vi "CalibrateImage.vi"() -> ()   [LabVIEW 2009]
uses:
  <vilib>/vision/NI_Vision_Development_Module.lvlib
panel:
  in  "Interpolation Type":u32(ring) items=["Zero Order", "Bi-Linear", "Quadratic", "Cubic Spline"]
  out "'input Image 2":T1(plugin-control)
  in  "Grid Descriptor":T2={"X Step"=1.0, "Y Step"=1.0, "Unit"=enum."Undefined", "Threshold Range"={"Lower value"=30.0, "Upper value"=96.0}} {"Threshold Range"."Upper value" format="%.2f"; "Threshold Range"."Lower value" format="%.2f"; "Y Step" format="%.2f"; "X Step" format="%.2f"}
  in  "Calibration Learn Setup":T4={"Distortion"=0, "Corrected Image Scaling"=0, "Corrected Image Learn ROI"=2, "Learn Error Map?"=FALSE, "Learn Correction Table?"=FALSE} {"Corrected Image Learn ROI" items=["Full Image ", "Calibration ROI", "ROI", "Calibration AND ROI", "Calibration OR ROI"]; "Corrected Image Scaling" items=["Scale to Preserve Area", "Scale to Fit"]; "Distortion" items=["Perspective", "Nonlinear"]}
  in  "Input Image Path":path=path "C:/Documents and Settings/ekolker/My Documents/OGRE/to be synched/camCal.JPG"
  out "'input Image":T1(plugin-control)
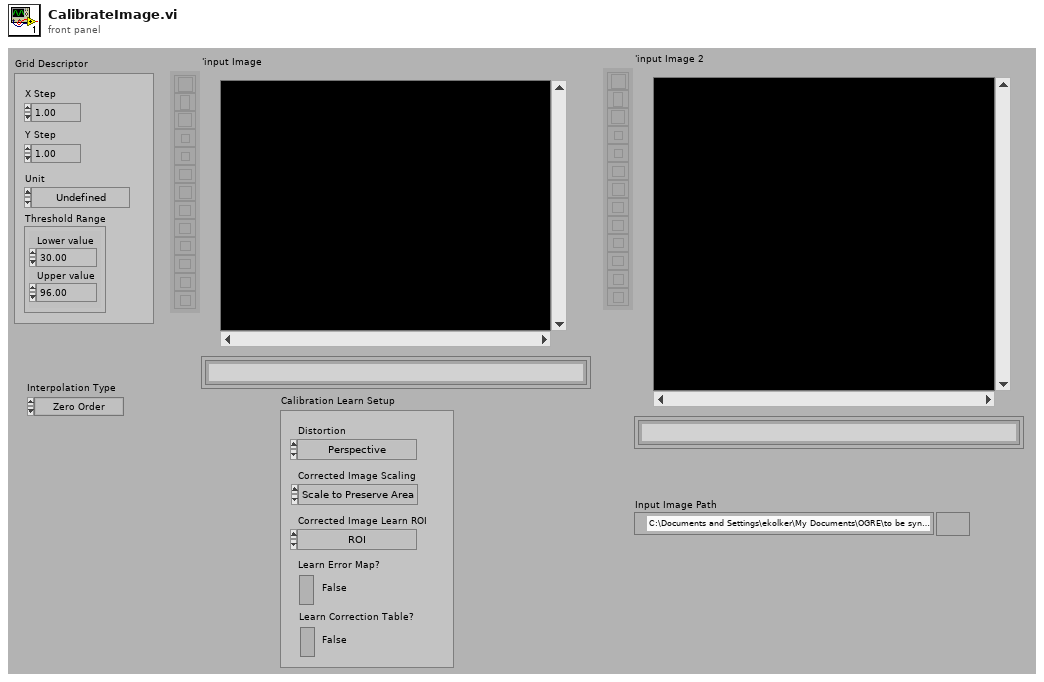
[diagram p1: front panel]
types:
  T1 = typedef "IMAQ Image.ctl" = refnum<image>
  T2 = typedef "Grid Descriptor" = cluster{"X Step":sgl, "Y Step":sgl, "Unit":T3, "Threshold Range":cluster{"Lower value":sgl, "Upper value":sgl}}
  T3 = typedef "Image Unit" = enum32{"Undefined", "Angström", "Micrometer", "Millimeter", "Centimeter", "Meter", "Kilometer", "Microinch", "Inch", "Feet", "Nautical miles", "Standard miles", "Steps"}
  T4 = cluster{"Distortion":u32, "Corrected Image Scaling":u32, "Corrected Image Learn ROI":u32, "Learn Error Map?":bool, "Learn Correction Table?":bool}
  T5 = typedef "Image Type" = u32
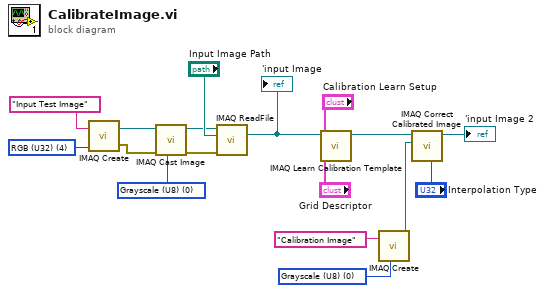
[diagram p0: block diagram]
diagram:
  w1 = T5 0 items=["Grayscale (U8)", "Grayscale (I16)", "Grayscale (SGL)", "Complex (CSG)", "RGB (U32)", "HSL (U32)", "RGB (U64)", "Grayscale (U16)"] ("Image Type")
  w14 = T5 0 items=["Grayscale (U8)", "Grayscale (I16)", "Grayscale (SGL)", "Complex (CSG)", "RGB (U32)", "HSL (U32)", "RGB (U64)", "Grayscale (U16)"] ("Image Type")
  w16 = T5 4 items=["Grayscale (U8)", "Grayscale (I16)", "Grayscale (SGL)", "Complex (CSG)", "RGB (U32)", "HSL (U32)", "RGB (U64)", "Grayscale (U16)"] ("Image Type")
  n1 = call "IMAQ Create"("Image Name"="Input Test Image", "Image Type"=w16) -> ("New Image"=w3:T1, "error out"=w11:errorcluster)  [unwired: 2 in, 1 out]
  n2 = call "IMAQ Cast Image"("Image Type"=w1, "Image Src"=w3) -> ("Image Dst Out"=w2:T1)  [unwired: 8 in, 1 out]
  n3 = call "IMAQ ReadFile"("File Path"="Input Image Path", "error in (no error)"=w11, "Image"=w2) -> ("Image Out"=w10:T1)  [unwired: 4 in, 4 out]
  "'input Image" <- w10
  n4 = call "IMAQ Learn Calibration Template"("Grid Descriptor"="Grid Descriptor", "Calibration Learn Setup"="Calibration Learn Setup", "Image"=w10) -> ("Calibrated Image"=w7:T1)  [unwired: 6 in, 2 out]
  n5 = call "IMAQ Create"("Image Name"="Calibration Image", "Image Type"=w14) -> ("New Image"=w6:T1)  [unwired: 2 in, 2 out]
  n6 = call "IMAQ Correct Calibrated Image"("Interpolation Type"="Interpolation Type", "Image Dst"=w6, "Image Src"=w7) -> ("Corrected Image"=→"'input Image 2":T1)  [unwired: 7 in, 1 out]
